vi "Write Speed.vi"(8 "error in (no error)":errorcluster, 10 "AxisSpeed":T1(array[cluster]), 11 "AxisCard in":refnum<class "AxisCard.lvclass">) -> (0 "error out":errorcluster, 3 "AxisCard out":refnum<class "AxisCard.lvclass">)   [LabVIEW 2019, in "AxisCard.lvclass"]
uses:
  AxisCard.lvclass
  AxisCard.lvclass/AxisCard.ctl
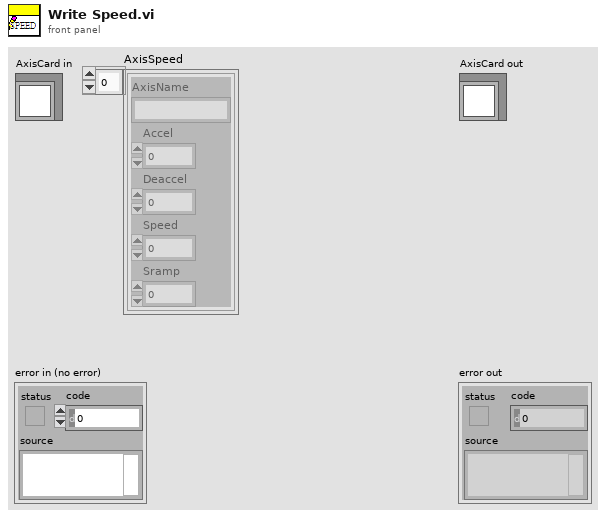
[diagram p1: front panel]
types:
  T1 = cluster{"AxisName":string, "Accel":dbl, "Deaccel":dbl, "Speed":dbl, "Sramp":dbl}[]
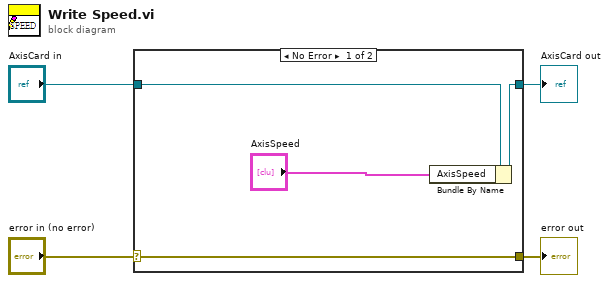
[diagram p0: block diagram]
diagram:
  n1 = case shown="No Error" "error in (no error)" {
    selector: "error in (no error)" -> [w8 w9]
    tunnel: [w8 w9] -> w3
    tunnel: [w6 w10] -> w1
    tunnel: "AxisCard in" -> [w7 w10]
    frame No Error {
      n2 = Bundle By Name(cluster=w7, "AxisSpeed"="AxisSpeed") -> (w6:refnum<class "AxisCard.lvclass">)
    }
    frame Error {
    }
  }
  "error out" <- w3
  "AxisCard out" <- w1
